vi "PID Derivative Control.vi"(0 "Temp In (deg C)":dbl format="%.2f", 7 "Control Parameters":T1={"Setpoint"=50.0, "Control Bandwidth"=4.0, "Integral Time"=30.0, "Int\nON"=TRUE, "Derivative Tme"=0.5, "Der\nON"=TRUE, "Settle Bandwidth"=1.0, "Settle Time"=30.0} {"Settle Time" step=1.0; "Settle Bandwidth" step=0.01; "Derivative Tme" step=0.01; "Integral Time" step=1.0; "Control Bandwidth" step=0.1; "Setpoint" step=0.1}, 9 "reset":bool, 11 "delta t":dbl format="%.2f") -> (8 "Derivative Power":dbl format="%.2f")   [LabVIEW 2019]
doc: "This is a Bug C(T) subVI.\n\nThis VI does the PID deriviative calculation.\n\nPaul K Dixon\nPhysics 3600\nCSUSB Physics"
uses:
  typedefs/PID control parameters.ctl
panel:
  # "PID\nDerivative\nPower\nControl"
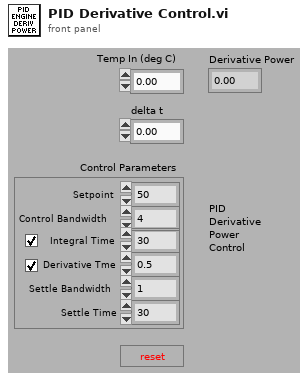
[diagram p1: front panel]
types:
  T1 = typedef "PID control parameters.ctl" = cluster{"Setpoint":dbl, "Control Bandwidth":dbl, "Integral Time":dbl, "Int\nON":bool, "Derivative Tme":dbl, "Der\nON":bool, "Settle Bandwidth":dbl, "Settle Time":dbl}
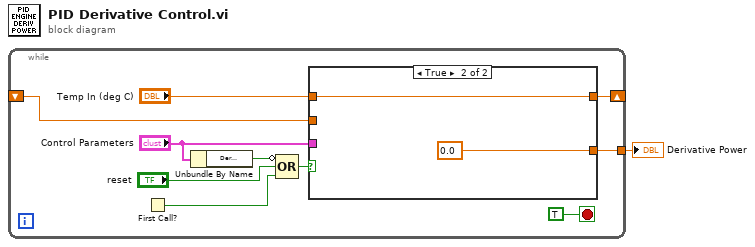
[diagram p0: block diagram]
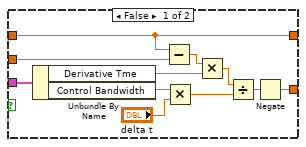
[diagram p2: hidden frame]
diagram:
  n1 = while {
    shift-left: _ -> [w5]
    shift-right: [w6] -> _
    tunnel: [w11] -> w1
    stop <- TRUE stop-if-true
    n2 = First Call?() -> (First Call?: T/F=w3:bool)
    n3 = Unbundle By Name("Control Parameters") -> ("Der\nON"=w2:bool)
    n4 = Compound Arithmetic op=OR(invert w2, "reset", w3) -> (w9:bool)
    n5 = case shown="True" w9 {
      tunnel: [w22 0.0] -> w11
      tunnel: "Control Parameters" -> [w21 _]
      tunnel: [w14 w23] -> w6
      tunnel: w5 -> [w17 _]
      tunnel: "Temp In (deg C)" -> [w14 w23]
      frame False {
        n6 = Unbundle By Name(w21) -> ("Derivative Tme"=w16:dbl, "Control Bandwidth"=w13:dbl)
        n7 = Subtract(x=w14, y=w17) -> (x-y=w15:dbl)
        n8 = Multiply(x=w13, y="delta t") -> (x*y=w19:dbl)
        n9 = Multiply(x=w15, y=w16) -> (x*y=w18:dbl)
        n10 = Divide(x=w18, y=w19) -> (x/y=w20:dbl)
        n11 = Negate(x=w20) -> (-x=w22:dbl)
      }
      frame True {
      }
    }
  }
  "Derivative Power" <- w1
